vi "BRig_FPGA_v3,91__PortC.vi"() -> ()   [LabVIEW 2014]
uses:
  <vilib>/rvi/Emulation/niFpgaGetClockAttributes.vi
  <vilib>/rvi/Emulation/niFpgaSctlEmulationGetInTimedLoop.vi
  <vilib>/rvi/Emulation/niFpgaEmulationReportErrorSimple.vi
  <vilib>/rvi/eio/common/nirviEmuTemplateMethod_errors.vi
  <vilib>/rvi/Emulation/niFpgaCriticalErrorInLSC.vi
  <vilib>/eio/EIONode/EIONode.xnode
panel:
  in  "L2Led_ON":bool
  in  "L1Led_ON":bool
  in  "Rising(F)_or_Falling(T)":bool
  in  "Solenoid_trig_R":bool
  in  "Solenoid_trig_L":bool
  in  "Solenoid_nTotal_R":u32=100
  in  "Solenoid_nTotal_L":u32=100
  in  "L2Led_Baseline":bool
  in  "L1Led_Baseline":bool
  in  "CueLed_Baseline":bool
  in  "I_allReward":bool
  in  "AnaOut_1":i16
  in  "CueLed_Event":bool
  in  "CueLed_nValley":u32=100
  in  "CueLed_nPeak":u32=100
  in  "LC_Event_l2":bool
  in  "LC_Laser_l2":bool
  in  "LC_nShutter_l2":u32=100
  in  "LC_nValley_l2":u32=100
  in  "LC_nPeak_l2":u32=100
  in  "LR_wrong_nDelay_l2":u32
  in  "LR_reward_nDelay_l2":u32
  in  "LR_wrong_nTotal_l2":u32=100
  in  "LR_reward_nTotal_l2":u32=100
  in  "LR_wrong_laser_l2":bool
  in  "LR_wrong_Event_l2":bool
  in  "LR_reward_Laser_l2":bool
  in  "LR_reward_Event_l2":bool
  out "AnaIn_1":i16
  out "AnaIn_0":i16
  out "timeTrial_count":u32
  in  "timeTrial_trig":bool
  in  "k1__counter_per_ms":u16=100 min=100 max=40000 step=1
  in  "LC_nShutter_l1":u32=100
  in  "AnaOut_0":i16
  in  "LC_nValley_l1":u32=100
  in  "LC_nPeak_l1":u32=100
  in  "LC_Event_l1":bool
  in  "LR_wrong_nTotal_l1":u32=100
  in  "LR_wrong_nDelay_l1":u32
  in  "LR_reward_nTotal_l1":u32=100
  in  "LR_reward_nDelay_l1":u32
  in  "LR_reward_Event_l1":bool
  in  "LR_wrong_Event_l1":bool
  out "SelectWrong":bool
  out "SelectReward":bool
  in  "LR_wrong_Laser_l1":bool
  in  "LR_reward_Laser_l1":bool
  in  "Left(F)_or_Right(T)":bool
  in  "ignoreWrong":bool
  in  "SelectionState":bool
  in  "LC_Laser_l1":bool
  in  "FPGA_Stop":bool
  in  "audioTrigger_L":bool
  in  "audioTrigger_R":bool
  in  "audioFreq_L_kHz":u8=14 min=1 max=14 step=1
  in  "audioAmp_L":u16=1 min=1 max=32767 step=1
  in  "audioFreq_R_kHz":u8=14 min=1 max=14 step=1
  in  "audioAmp_R":u16=1 min=1 max=32767 step=1
  in  "A3_SL":bool
  in  "A1_SR":bool
  in  "Counts_Reset":bool
  out "A4_LickR":u32
  out "A2_LickL":u32
  in  "A6_Act":bool
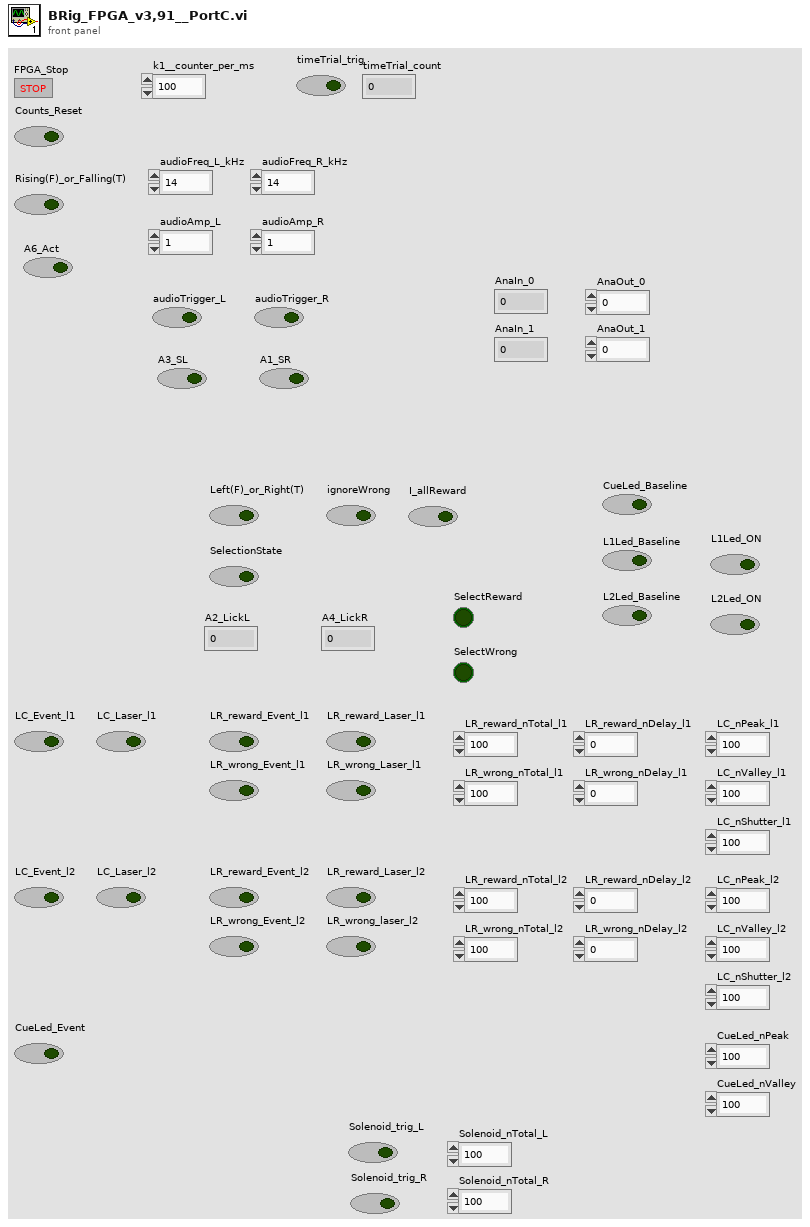
[diagram p1: front panel]
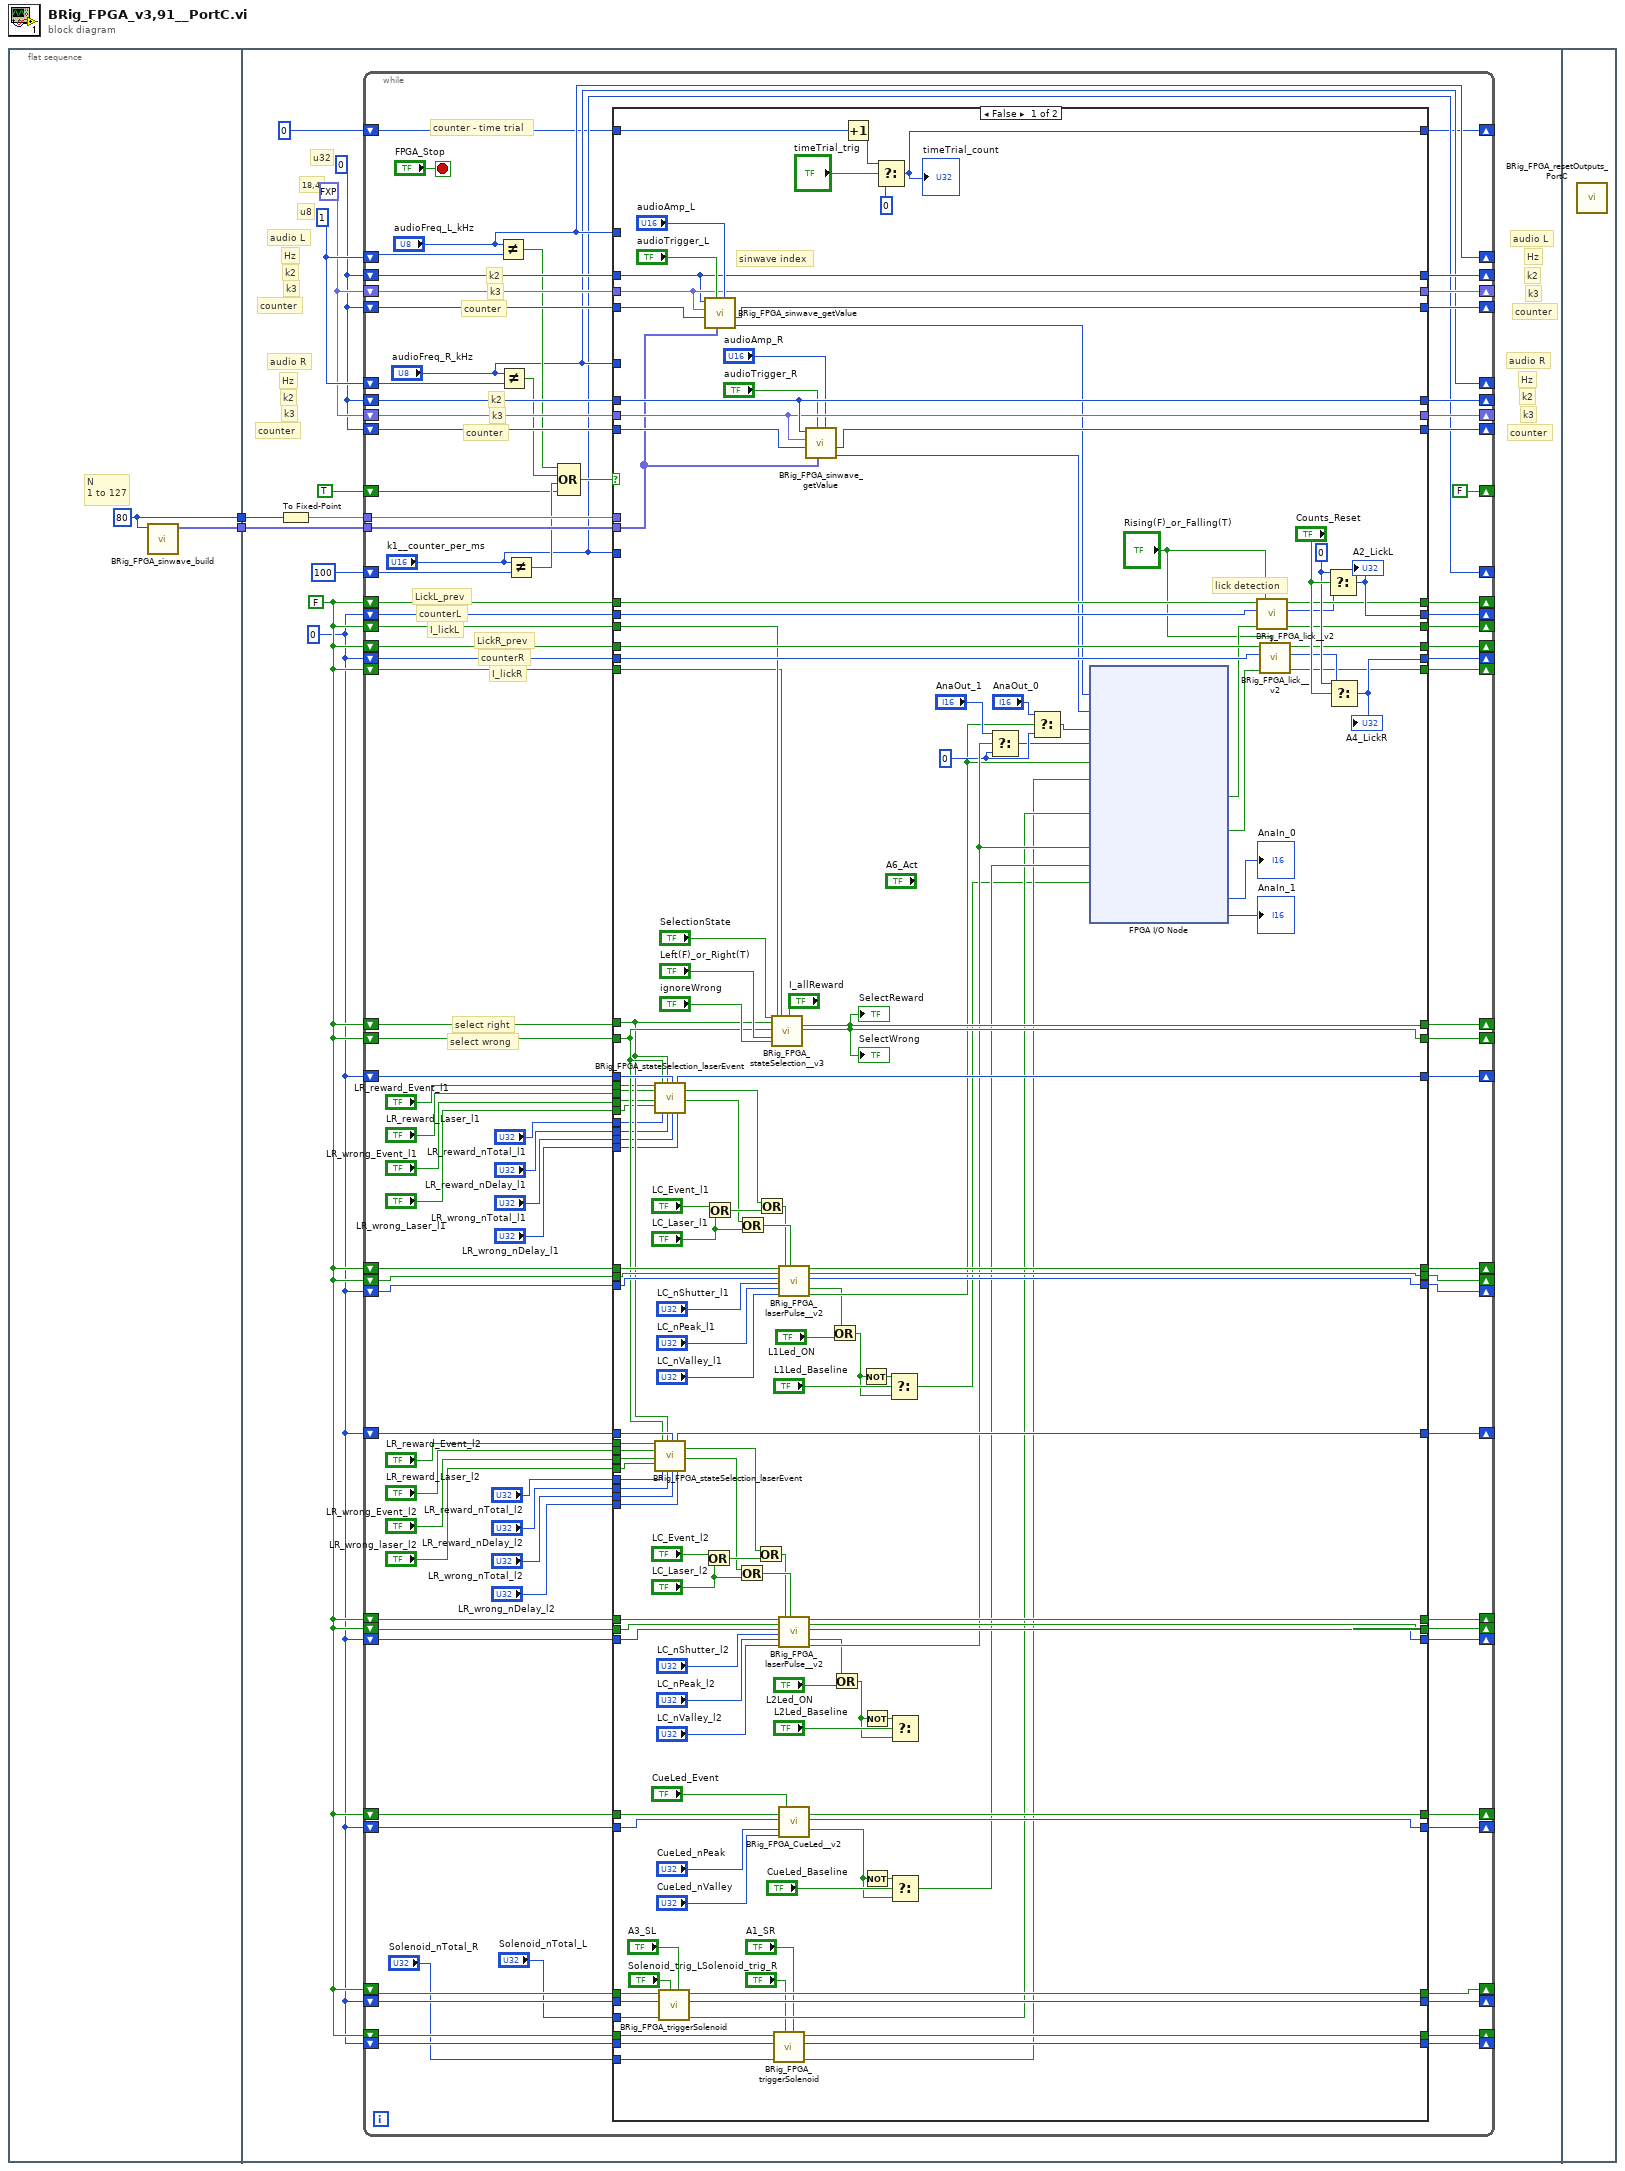
[diagram p0: block diagram]
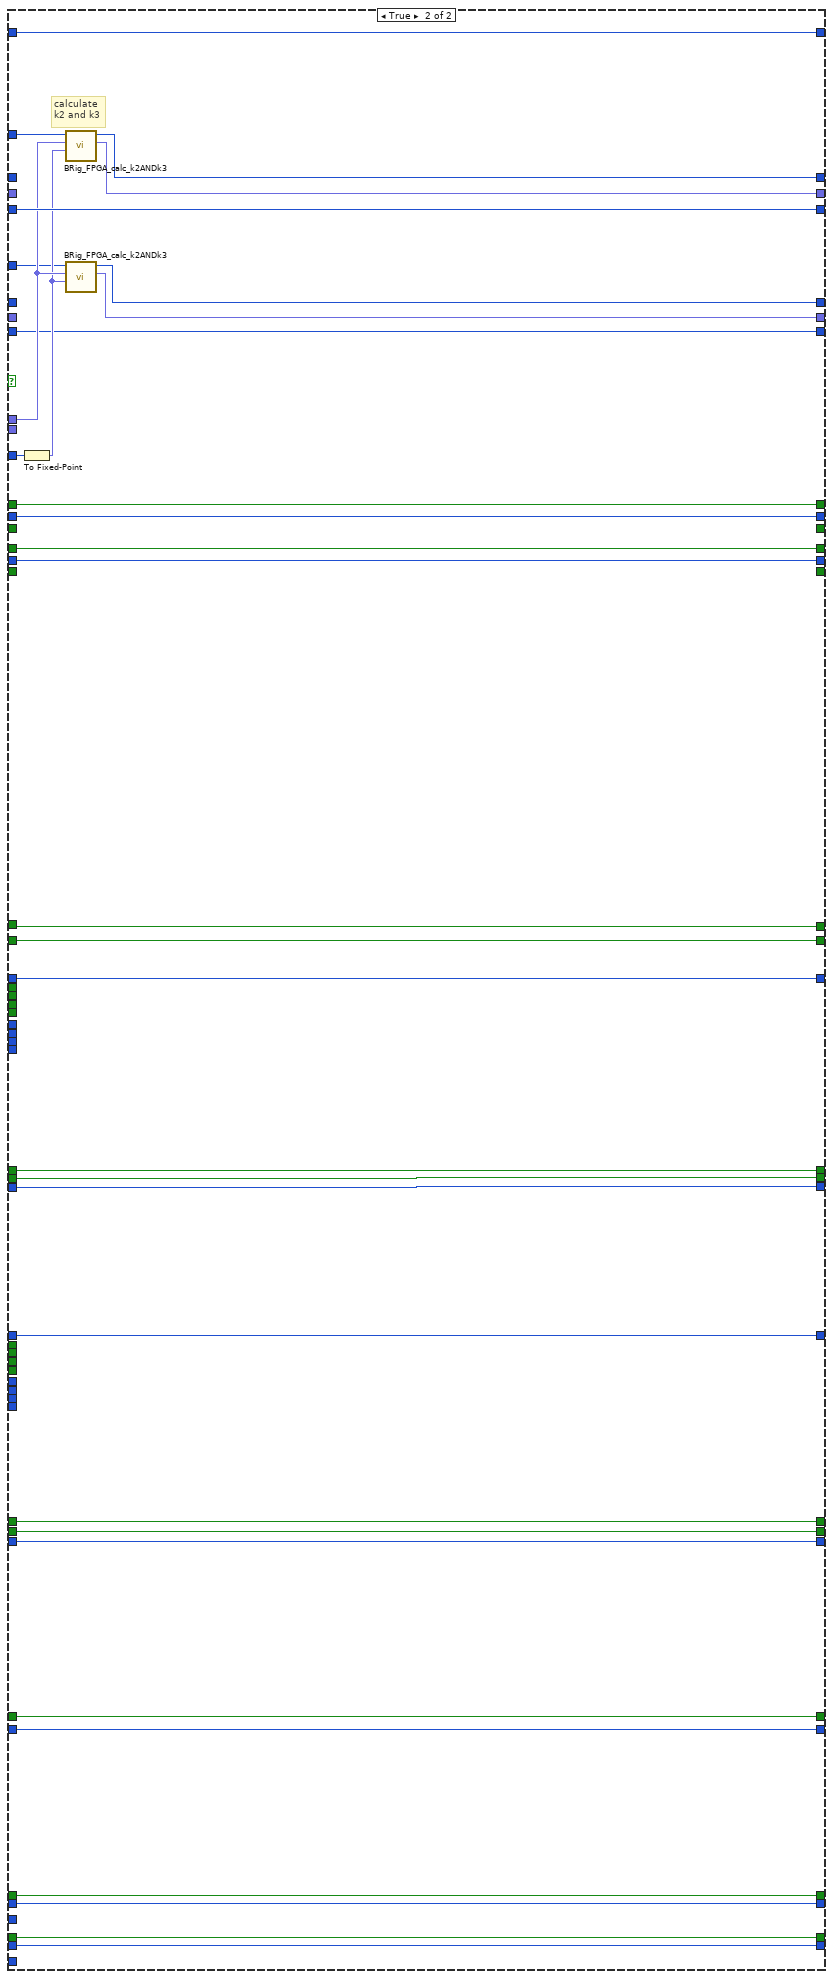
[diagram p2: hidden frame]
diagram:
  n1 = flat-sequence {
    tunnel: [w4] -> w2
    tunnel: [w3] -> w1
    tunnel: w2 -> [w15]
    tunnel: w1 -> [w14]
    frame #0 {
      w3 = 80 ("dimension size")
      # "N\n1 to 127"
      n2 = call "BRig_FPGA_sinwave_build.vi"("input_Npts"=w3) -> ("output_array_sin"=w4:fxp<+/-,16,2>[])  [unwired: 10 in]
    }
    frame #1 {
      w5 = u32 0
      w6 = FALSE
      w10 = u32 0
      w11 = fxp<+,18,4> 0.0
      w12 = u8 1
      # "counter"
      # "k3"
      # "k2"
      # "counter"
      # "k3"
      # "k2"
      # "counter"
      # "counter"
      # "u32"
      # "k3"
      # "k2"
      # "k3"
      # "18,4"
      # "u8"
      # "Hz"
      # "Hz"
      # "audio R"
      # "audio L"
      # "Hz"
      # "k2"
      # "Hz"
      # "audio R"
      # "audio L"
      n3 = To Fixed-Point(number=w14) -> (fixed-point=w13:fxp<+,7,7>)  [unwired: 1 in]
      n4 = while {
        shift-right: ["audioFreq_L_kHz"] -> _
        shift-left: w12 -> [w106]
        shift-right: [w100] -> _
        shift-left: w10 -> [w104]
        shift-right: ["audioFreq_R_kHz"] -> _
        shift-left: w12 -> [w96]
        tunnel: w15 -> [w103]
        tunnel: w13 -> [w102]
        shift-right: [w99] -> _
        shift-left: w11 -> [w101]
        shift-right: [w97] -> _
        shift-left: w10 -> [w98]
        shift-right: [w94] -> _
        shift-left: w10 -> [w95]
        shift-right: [w92] -> _
        shift-left: w11 -> [w93]
        shift-right: [w90] -> _
        shift-left: w10 -> [w91]
        shift-right: ["k1__counter_per_ms"] -> _
        shift-left: u16 100 ("y") -> [w89]
        shift-right: [FALSE] -> _
        shift-left: TRUE -> [w84]
        shift-right: [w77] -> _
        shift-left: w6 -> [w79]
        shift-right: [w76] -> _
        shift-left: w6 -> [w78]
        shift-right: [w74] -> _
        shift-left: w5 -> [w75]
        shift-right: [w72] -> _
        shift-left: w5 -> [w73]
        shift-right: [w69] -> _
        shift-left: w6 -> [w71]
        shift-right: [w68] -> _
        shift-left: w6 -> [w70]
        shift-right: [w66] -> _
        shift-left: w6 -> [w67]
        shift-right: [w64] -> _
        shift-left: w6 -> [w65]
        shift-right: [w62] -> _
        shift-left: u32 0 -> [w63]
        shift-right: [w60] -> _
        shift-left: w5 -> [w61]
        shift-right: [w59] -> _
        shift-left: w6 -> [w56]
        shift-right: [w58] -> _
        shift-left: w6 -> [w55]
        shift-right: [w57] -> _
        shift-left: w5 -> [w54]
        shift-right: [w52] -> _
        shift-left: w5 -> [w53]
        shift-right: [w51] -> _
        shift-left: w6 -> [w48]
        shift-right: [w50] -> _
        shift-left: w6 -> [w47]
        shift-right: [w49] -> _
        shift-left: w5 -> [w46]
        shift-right: [w45] -> _
        shift-left: w6 -> [w43]
        shift-right: [w44] -> _
        shift-left: w5 -> [w42]
        shift-right: [w24] -> _
        shift-left: w5 -> [w25]
        shift-right: [w21] -> _
        shift-left: w6 -> [w23]
        shift-right: [w18] -> _
        shift-left: w6 -> [w20]
        shift-right: [w17] -> _
        shift-left: w5 -> [w19]
        stop <- "FPGA_Stop" stop-if-true
        # "counter"
        # "k3"
        # "k2"
        # "counter"
        # "k3"
        # "k2"
        # "counter - time trial"
        # "I_lickR"
        # "counterR"
        # "LickR_prev"
        # "I_lickL"
        # "counterL"
        # "LickL_prev"
        # "select wrong"
        # "select right"
        n5 = Not Equal?(x="audioFreq_L_kHz", y=w106) -> (x != y?=w88:bool)
        n6 = Not Equal?(x="audioFreq_R_kHz", y=w96) -> (x != y?=w87:bool)
        n7 = Not Equal?(x="k1__counter_per_ms", y=w89) -> (x != y?=w85:bool)
        n8 = Compound Arithmetic op=OR(w88, w87, w85, w84) -> (w86:bool)
        n9 = case shown="False" w86 {
          tunnel: w104 -> [w237 _]
          tunnel: "audioFreq_L_kHz" -> [_ w283]
          tunnel: w103 -> [w230 _]
          tunnel: w102 -> [_ w279]
          tunnel: "k1__counter_per_ms" -> [_ w284]
          tunnel: w101 -> [w238 _]
          tunnel: [w237 w282] -> w100
          tunnel: [w238 w281] -> w99
          tunnel: w98 -> [w242 w280]
          tunnel: [w239 w280] -> w97
          tunnel: w95 -> [w234 _]
          tunnel: [w234 w275] -> w94
          tunnel: w93 -> [w233 _]
          tunnel: [w233 w276] -> w92
          tunnel: w91 -> [w236 w274]
          tunnel: "audioFreq_R_kHz" -> [_ w277]
          tunnel: [w235 w274] -> w90
          tunnel: w79 -> [w225 w273]
          tunnel: w78 -> [w224 w272]
          tunnel: [w229 w273] -> w77
          tunnel: [w222 w272] -> w76
          tunnel: w75 -> [w226 w271]
          tunnel: [w252 w271] -> w74
          tunnel: w73 -> [w223 w270]
          tunnel: [w249 w270] -> w72
          tunnel: w71 -> [w176 w269]
          tunnel: w70 -> [w177 w268]
          tunnel: [w196 w269] -> w69
          tunnel: [w245 w268] -> w68
          tunnel: [w215 w265] -> w59
          tunnel: [w216 w264] -> w58
          tunnel: [w217 w263] -> w57
          tunnel: w67 -> [w219 _]
          tunnel: [w228 _] -> w66
          tunnel: w65 -> [w218 _]
          tunnel: [w220 _] -> w64
          tunnel: w63 -> [w207 w267]
          tunnel: [w204 w267] -> w62
          tunnel: w61 -> [w195 w266]
          tunnel: [w194 w266] -> w60
          tunnel: w56 -> [w193 w265]
          tunnel: w55 -> [w192 w264]
          tunnel: w54 -> [w191 w263]
          tunnel: w53 -> [w179 w262]
          tunnel: [w178 w262] -> w52
          tunnel: [w174 w261] -> w51
          tunnel: [w173 w260] -> w50
          tunnel: [w172 w259] -> w49
          tunnel: w48 -> [w171 w261]
          tunnel: w47 -> [w170 w260]
          tunnel: w46 -> [w169 w259]
          tunnel: [w166 w258] -> w45
          tunnel: [w165 w257] -> w44
          tunnel: w43 -> [w164 w258]
          tunnel: w42 -> [w163 w257]
          tunnel: "LR_reward_Event_l1" -> [w146 _]
          tunnel: "LR_reward_Laser_l1" -> [w145 _]
          tunnel: "LR_wrong_Event_l1" -> [w144 _]
          tunnel: "LR_wrong_Laser_l1" -> [w143 _]
          tunnel: "LR_reward_nTotal_l1" -> [w142 _]
          tunnel: "LR_reward_nDelay_l1" -> [w141 _]
          tunnel: "LR_wrong_nTotal_l1" -> [w140 _]
          tunnel: "LR_wrong_nDelay_l1" -> [w139 _]
          tunnel: "LR_reward_Event_l2" -> [w138 _]
          tunnel: "LR_reward_Laser_l2" -> [w137 _]
          tunnel: "LR_wrong_Event_l2" -> [w136 _]
          tunnel: "LR_wrong_laser_l2" -> [w135 _]
          tunnel: "LR_reward_nTotal_l2" -> [w134 _]
          tunnel: "LR_reward_nDelay_l2" -> [w133 _]
          tunnel: "LR_wrong_nTotal_l2" -> [w132 _]
          tunnel: "LR_wrong_nDelay_l2" -> [w131 _]
          tunnel: w25 -> [w130 w256]
          tunnel: [w125 w256] -> w24
          tunnel: w23 -> [w129 w255]
          tunnel: "Solenoid_nTotal_L" -> [w128 _]
          tunnel: [w124 w255] -> w21
          tunnel: w20 -> [w120 w254]
          tunnel: w19 -> [w119 w253]
          tunnel: [w118 w254] -> w18
          tunnel: [w117 w253] -> w17
          tunnel: "Solenoid_nTotal_R" -> [w116 _]
          frame False {
            w159 = i16 0 ("f")
            w250 = u32 0 ("t")
            # "sinwave index"
            # "lick detection"
            n10 = call "BRig_FPGA_stateSelection_laserEvent.vi"("I_LR_reward"=w146, "I_LR_reward_laser"=w145, "I_LR_wrong"=w144, "I_LR_wrong_laser"=w143, "I_selectWrong"=w177, "laser_reward_nTotal"=w142, "I_selectReward"=w176, "laser_reward_nDelay"=w141, "counter"=w195, "laser_wrong_nTotal"=w140, "laser_wrong_nDelay"=w139) -> ("output_counter"=w194:u32, "output_I_laserEvent"=w190:bool, "output_I_laserOn"=w189:bool)  [unwired: 6 in]
            n11 = call "BRig_FPGA_stateSelection_laserEvent.vi"("I_LR_reward"=w138, "I_LR_reward_laser"=w137, "I_LR_wrong"=w136, "I_LR_wrong_laser"=w135, "I_selectWrong"=w177, "laser_reward_nTotal"=w134, "I_selectReward"=w176, "laser_reward_nDelay"=w133, "counter"=w179, "laser_wrong_nTotal"=w132, "laser_wrong_nDelay"=w131) -> ("output_counter"=w178:u32, "output_I_laserEvent"=w175:bool, "output_I_laserOn"=w180:bool)  [unwired: 6 in]
            n12 = call "BRig_FPGA_triggerSolenoid.vi"("input_Solenoid_MTrig"="A3_SL", "input_Solenoid_trig"="Solenoid_trig_L", "input_threshold"=w128, "input_counter"=w130, "input_trig"=w129) -> ("output_Solenoid_OnOff"=w123:bool, "output_counter"=w125:u32, "output_trig"=w124:bool)  [unwired: 4 in]
            n13 = Or(x="LC_Event_l2", y="LC_Laser_l2") -> (x .or. y?=w184:bool)
            n14 = call "BRig_FPGA_sinwave_getValue.vi"("audioAmp"="audioAmp_L", "sinwave"=w230, "audioTrigger"="audioTrigger_L", "counter"=w242, "k3"=w238, "k2"=w237) -> ("output_audioValue"=w202:i16, "output_counter"=w239:u32)  [unwired: 4 in]
            n15 = Or(x="LC_Event_l1", y="LC_Laser_l1") -> (x .or. y?=w211:bool)
            n16 = Or(x=w180, y="LC_Laser_l2") -> (x .or. y?=w182:bool)
            n17 = Or(x=w189, y="LC_Laser_l1") -> (x .or. y?=w209:bool)
            n18 = Or(x=w175, y=w184) -> (x .or. y?=w181:bool)
            n19 = Or(x=w190, y=w211) -> (x .or. y?=w208:bool)
            n20 = call "BRig_FPGA_stateSelection__v3.vi"("I_selectionState"="SelectionState", "I_selectRight"=w176, "I_selectWrong"=w177, "I_Left(F)_or_Right(T)"="Left(F)_or_Right(T)", "I_ignoreWrong"="ignoreWrong", "I_lickL"=w219, "I_lickR"=w218, "I_allReward"="I_allReward") -> ("output__I_selectRight"=w196:bool, "output__I_selectWrong"=w245:bool)  [unwired: 18 in]
            "SelectWrong" <- w245
            "SelectReward" <- w196
            n21 = call "BRig_FPGA_triggerSolenoid.vi"("input_Solenoid_MTrig"="A1_SR", "input_Solenoid_trig"="Solenoid_trig_R", "input_threshold"=w116, "input_counter"=w119, "input_trig"=w120) -> ("output_Solenoid_OnOff"=w115:bool, "output_counter"=w117:u32, "output_trig"=w118:bool)  [unwired: 4 in]
            n22 = call "BRig_FPGA_laserPulse__v2.vi"("I_shutter"=w193, "I_peak"=w192, "count"=w191, "laser_Nshutter"="LC_nShutter_l1", "laser_Npeak"="LC_nPeak_l1", "laser_Nvalley"="LC_nValley_l1", "I_laserEvent"=w208, "I_laser"=w209) -> ("output_I_shutter"=w215:bool, "output_I_peak"=w216:bool, "output_count"=w217:u32, "output_led"=w111:bool, "output_laser"=w157:bool)  [unwired: 6 in, 1 out]
            n23 = call "BRig_FPGA_laserPulse__v2.vi"("I_shutter"=w171, "I_peak"=w170, "count"=w169, "laser_Nshutter"="LC_nShutter_l2", "laser_Npeak"="LC_nPeak_l2", "laser_Nvalley"="LC_nValley_l2", "I_laserEvent"=w181, "I_laser"=w182) -> ("output_I_shutter"=w174:bool, "output_I_peak"=w173:bool, "output_count"=w172:u32, "output_led"=w108:bool, "output_laser"=w160:bool)  [unwired: 6 in, 1 out]
            n24 = call "BRig_FPGA_CueLed__v2.vi"("I_peak"=w164, "count"=w163, "laser_Npeak"="CueLed_nPeak", "laser_Nvalley"="CueLed_nValley", "I_CueLed_Event"="CueLed_Event") -> ("output_I_peak"=w166:bool, "output_count"=w165:u32, "output_led"=w151:bool)  [unwired: 12 in]
            n25 = call "BRig_FPGA_sinwave_getValue.vi"("audioAmp"="audioAmp_R", "sinwave"=w230, "audioTrigger"="audioTrigger_R", "counter"=w236, "k3"=w233, "k2"=w234) -> ("output_audioValue"=w201:i16, "output_counter"=w235:u32)  [unwired: 4 in]
            n26 = Or(x=w111, y="L1Led_ON") -> (x .or. y?=w110:bool)
            n27 = Or(x=w108, y="L2Led_ON") -> (x .or. y?=w107:bool)
            n28 = Increment(x=w207) -> (x+1=w206:u32)
            n29 = Not(x=w110) -> (.not. x?=w150:bool)
            n30 = Not(x=w107) -> (.not. x?=w148:bool)
            n31 = Not(x=w151) -> (.not. x?=w153:bool)
            n32 = Select(t=w206, s="timeTrial_trig", f=u32 0) -> (s? t:f=w204:u32)
            "timeTrial_count" <- w204
            n33 = Select(t=w150, s="L1Led_Baseline", f=w110) -> (s? t:f=w113:bool)
            n34 = Select(t=w148, s="L2Led_Baseline", f=w107) -> ()  [unwired: 1 out]
            n35 = Select(t=w153, s="CueLed_Baseline", f=w151) -> (s? t:f=w154:bool)
            n36 = Select(t="AnaOut_1", s=w160, f=w159) -> (s? t:f=w156:i16)
            n37 = Select(t="AnaOut_0", s=w157, f=w159) -> (s? t:f=w161:i16)
            n38 = xnode "FPGA I/O Node"("AudioOut/Left"=w202, "AudioOut/Right"=w201, "ConnectorC/AO0"=w161, "ConnectorC/AO1"=w156, "ConnectorC/DIO0"=w157, "ConnectorC/DIO1"=w115, "ConnectorC/DIO3"=w123, "ConnectorC/DIO5"=w160, "ConnectorC/DIO6"=w154, "ConnectorC/DIO7"=w113) -> ("ConnectorC/DIO2"=w200:bool, "ConnectorC/DIO4"=w199:bool, "ConnectorC/AI0"=→"AnaIn_0":i16, "ConnectorC/AI1"=→"AnaIn_1":i16)  [unwired: 14 in, 14 out]
            n39 = call "BRig_FPGA_lick__v2.vi"("Rising(F)_or_Falling(T)"="Rising(F)_or_Falling(T)", "I_stateDetector_new"=w200, "counter"=w226, "I_stateDetector_prev"=w225) -> ("output_I_lick"=w228:bool, "output_counter"=w227:u32, "output_I_stateDetector_prev"=w229:bool)  [unwired: 5 in]
            n40 = call "BRig_FPGA_lick__v2.vi"("Rising(F)_or_Falling(T)"="Rising(F)_or_Falling(T)", "I_stateDetector_new"=w199, "counter"=w223, "I_stateDetector_prev"=w224) -> ("output_I_lick"=w220:bool, "output_counter"=w221:u32, "output_I_stateDetector_prev"=w222:bool)  [unwired: 5 in]
            n41 = Select(t=w250, s="Counts_Reset", f=w227) -> (s? t:f=w252:u32)
            "A2_LickL" <- w252
            n42 = Select(t=w250, s="Counts_Reset", f=w221) -> (s? t:f=w249:u32)
            "A4_LickR" <- w249
          }
          frame True {
            # "calculate\nk2 and k3"
            n43 = To Fixed-Point(number=w284) -> (fixed-point=w278:fxp<+,16,16>)  [unwired: 1 in]
            n44 = call "BRig_FPGA_calc_k2ANDk3.vi"("input_k1[count/ms]"=w278, "input_Npts"=w279, "input_freq[kHz]"=w283) -> ("output_k3"=w281:fxp<+,18,4>, "output_k2"=w282:u32)  [unwired: 7 in]
            n45 = call "BRig_FPGA_calc_k2ANDk3.vi"("input_k1[count/ms]"=w278, "input_Npts"=w279, "input_freq[kHz]"=w277) -> ("output_k3"=w276:fxp<+,18,4>, "output_k2"=w275:u32)  [unwired: 7 in]
          }
        }
      }
    }
    frame #2 {
      n46 = call "BRig_FPGA_resetOutputs_PortC.vi"() -> ()  [unwired: 12 in]
    }
  }
